vi "Pair string Array.vi"(0 "Flat Array":string[](array[string])) -> (1 "Concatenated Strings":string[](array[string]), 2 "Extra Data":T1)   [LabVIEW 2016]
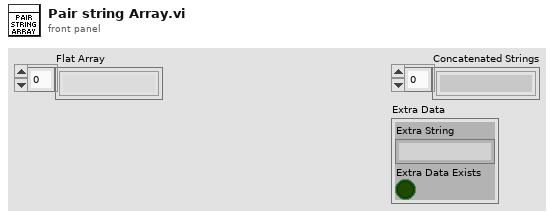
[diagram p1: front panel]
types:
  T1 = cluster{"Extra String":string, "Extra Data Exists":bool}
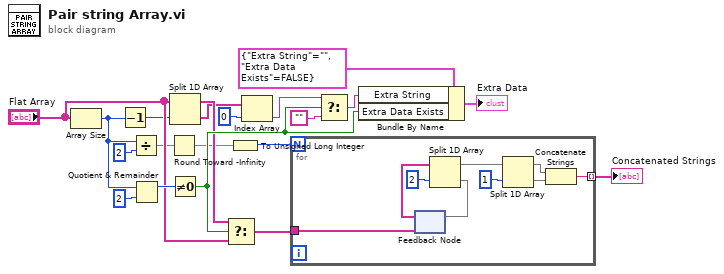
[diagram p0: block diagram]
diagram:
  n1 = Array Size(array="Flat Array") -> (size(s)=w11:i32)
  n2 = Decrement(x=w11) -> (x-1=w10:i32)
  n3 = Divide(x=w11, y=2) -> (x/y=w8:dbl)
  n4 = Quotient & Remainder(x=w11, y=2) -> (x-y*floor(x/y)=w17:i32)  [unwired: 1 out]
  n5 = Round Toward -Infinity(1:w8) -> (0:w7:dbl)
  n6 = Split 1D Array(array="Flat Array", index=w10) -> (first subarray=w9:string[], second subarray=w4:string[])
  n7 = Not Equal To 0?(x=w17) -> (x != 0?=w13:bool)
  n8 = Select(t=w9, s=w13, f="Flat Array") -> (s? t:f=w16:string[])
  n9 = To Unsigned Long Integer(number=w7) -> (unsigned 32bit integer=w19:u32)
  n10 = Index Array(array=w4, index=0) -> (element=w2:string)
  n11 = for {
    N: w19 -> [_]
    tunnel: w16 -> [w26]
    tunnel: [w21] -> w14 mode=indexing
    n12 = feedback #1(w26) -> (w28:string[])
    n13 = Split 1D Array(array=w28, index=2) -> (first subarray=w25:string[], second subarray=w27:string[])
    n14 = feedback-in #1(w27) -> ()
    n15 = Split 1D Array(array=w25, index=1) -> (first subarray=w23:string[], second subarray=w22:string[])
    n16 = Concatenate Strings(w23, w22) -> (w21:string)
  }
  "Concatenated Strings" <- w14
  n17 = Select(t=w2, s=w13, f="") -> (s? t:f=w5:string)
  n18 = Bundle By Name(cluster=T1 {"Extra String"="", "Extra Data Exists"=FALSE} ("input cluster"), "Extra String"=w5, "Extra Data Exists"=w13) -> (→"Extra Data":T1)
